vi "FreqtoNote.vi"(2 "Freq meas":dbl) -> (5 "Note":string, 6 "Half steps":i32, 7 "OctaveDn":i32, 8 "NotesUp":i32)   [LabVIEW 2015]
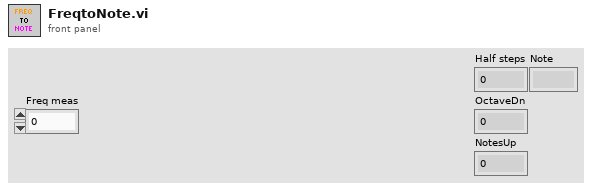
[diagram p1: front panel]
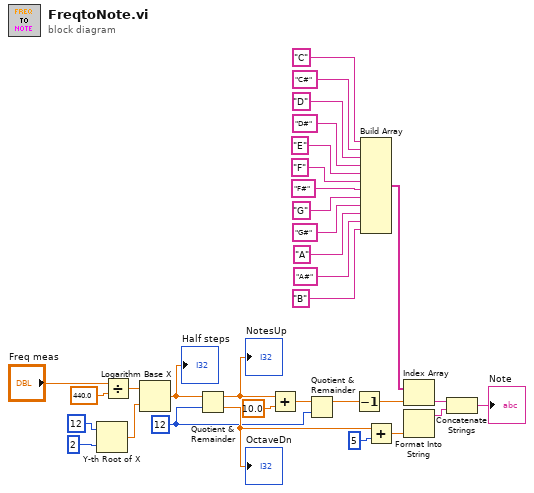
[diagram p0: block diagram]
diagram:
  w8 = 12
  n1 = Y-th Root of X(1:2, 2:12) -> (0:w27:dbl)
  n2 = Divide(x="Freq meas", y=440.0 ("Freq const")) -> (x/y=w30:dbl)
  n3 = Logarithm Base X(1:w27, 2:w30) -> (0:w26:dbl)
  "Half steps" <- w26
  n4 = Quotient & Remainder(x=w26, y=w8) -> (x-y*floor(x/y)=w10:dbl, floor(x/y)=w12:dbl)
  "OctaveDn" <- w12
  "NotesUp" <- w10
  n5 = Add(x=w10, y=10.0) -> (x+y=w7:dbl)
  n6 = Quotient & Remainder(x=w7, y=w8) -> (x-y*floor(x/y)=w2:dbl)  [unwired: 1 out]
  n7 = Decrement(x=w2) -> (x-1=w1:dbl)
  n8 = Build Array("C", "C#", "D", "D#", "E", "F", "F#", "G", "G#", "A", "A#", "B") -> (w9:string[])
  n9 = Add(x=w12, y=5) -> (x+y=w6:dbl)
  n10 = Index Array(array=w9, index=w1) -> (element=w4:string)
  n11 = Format Into String(w6) -> (resulting string=w5:string)  [unwired: 3 in, 1 out]
  n12 = Concatenate Strings(w4, w5) -> (→"Note":string)
